vi "Ignition.vi"(7 "Log File Refnum in":refnum<file>, 8 "error in":errorcluster, 9 "UI Data in":T2, 10 "Handshake Notifier in":refnum<notifier>, 11 "Message Queues in":T1) -> (0 "error out":errorcluster, 1 "UI Data out":T2, 2 "Handshake Notifier out":refnum<notifier>, 3 "Message Queues out":T1, 5 "Log File Refnum out":refnum<file>)   [LabVIEW 2014, in "Controller.lvlib"]
doc: "Light the pilot for the boiler."
uses:
  Controller.lvlib
  support/Boiler System Globals.vi
  controls/MHL Status.ctl
  support/Message Queue/Message Cluster.ctl
  support/Message Queue/All Message Queues.ctl
  controls/MHL UI Data.ctl
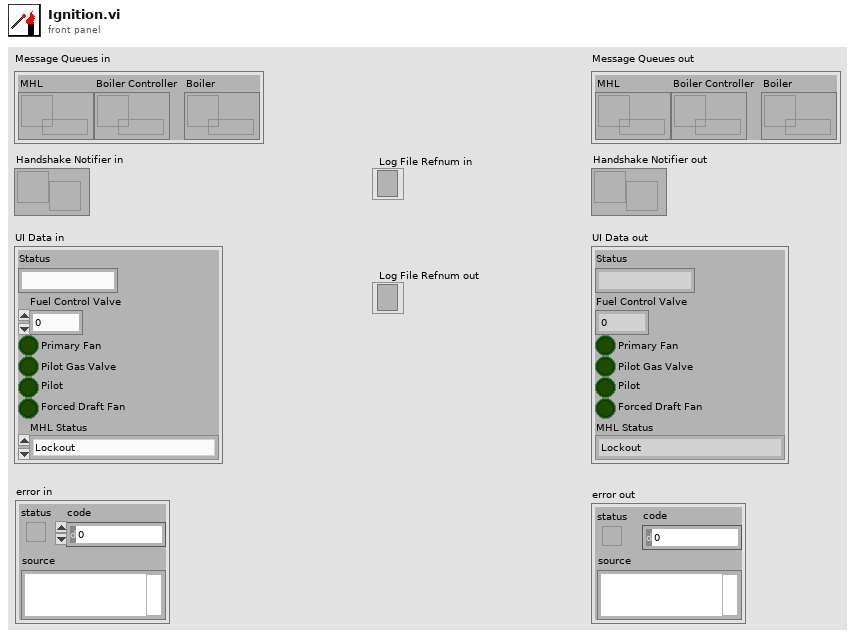
[diagram p1: front panel]
types:
  T1 = typedef "Message Queue.lvlib/All Message Queues.ctl" = cluster{"MHL":refnum<queue>, "Boiler Controller":refnum<queue>, "Boiler":refnum<queue>}
  T2 = typedef "MHL UI Data.ctl" = cluster{"Status":string, "Fuel Control Valve":u32, "Primary Fan":bool, "Pilot Gas Valve":bool, "Pilot":bool, "Forced Draft Fan":bool, "MHL Status":T3}
  T3 = typedef "MHL Status.ctl" = enum16{"Lockout", "Ready", "Pre-Purge", "Pre-Purge Complete", "Pilot On", "Boiler Running", "Shutdown", "Purge"}
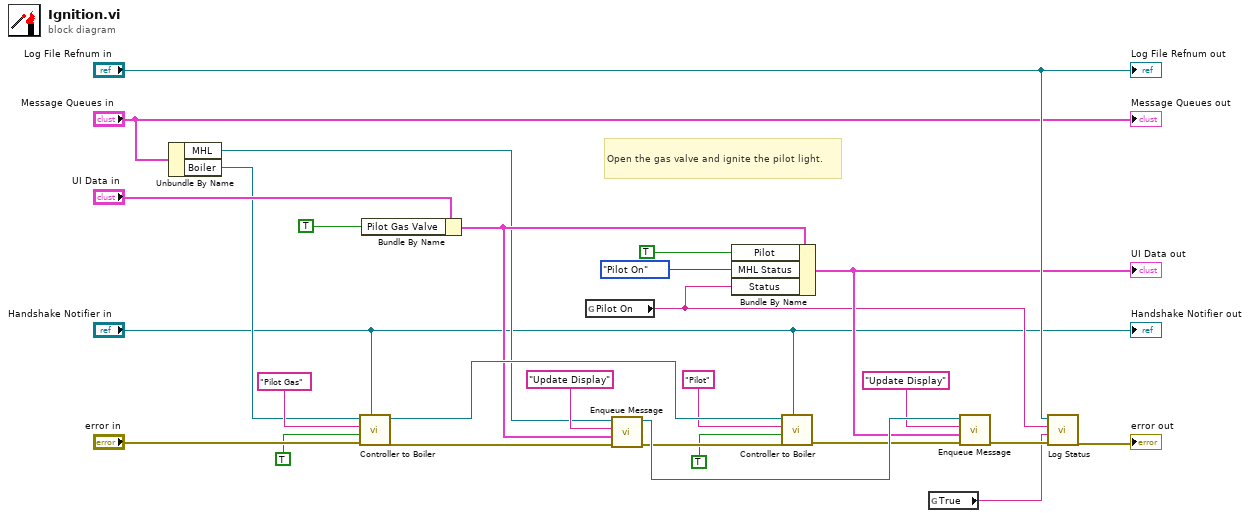
[diagram p0: block diagram]
diagram:
  # "Open the gas valve and ignite the pilot light."
  n1 = Unbundle By Name("Message Queues in") -> ("MHL"=w7:refnum<queue>, "Boiler"=w6:refnum<queue>)
  n2 = call "Controller to Boiler.vi"("Notifier"="Handshake Notifier in", "error in"="error in", "Message Data"=TRUE, "Message"="Pilot Gas", "Boiler Queue in"=w6) -> ("error out"=w22:errorcluster, "Queue out"=w26:refnum<queue>)  [unwired: 4 in, 1 out]
  n3 = Bundle By Name(cluster="UI Data in", "Pilot Gas Valve"=TRUE ("Natural Gas Valve")) -> (w25:T2)
  n4 = global read "Boiler System Globals.vi" "Pilot On"() -> (w4:string)
  n5 = call "Enqueue Message.vi"("error in (no error)"=w22, "Message Data"=w25, "Message"="Update Display", "Message Queue"=w7) -> ("error out"=w21:errorcluster, "dup Message Queue"=w23:refnum<queue>)  [unwired: 6 in]
  n6 = Bundle By Name(cluster=w25, "Pilot"=TRUE, "MHL Status"=MHL_Status."Pilot On", "Status"=w4) -> (w14:T2)
  "UI Data out" <- w14
  n7 = call "Controller to Boiler.vi"("Notifier"="Handshake Notifier in", "error in"=w21, "Message Data"=TRUE, "Message"="Pilot", "Boiler Queue in"=w26) -> ("error out"=w18:errorcluster)  [unwired: 4 in, 2 out]
  n8 = global read "Boiler System Globals.vi" "True"() -> (w3:string)
  n9 = call "Enqueue Message.vi"("error in (no error)"=w18, "Message Data"=w14, "Message"="Update Display", "Message Queue"=w23) -> ("error out"=w9:errorcluster)  [unwired: 6 in, 1 out]
  n10 = call "Log Status.vi"("error in"=w9, "Event Data String (-)"=w3, "Event String"=w4, "Log File Refnum In"="Log File Refnum in") -> ("error out"=→"error out":errorcluster)  [unwired: 6 in, 1 out]
  "Log File Refnum out" <- "Log File Refnum in"
  "Message Queues out" <- "Message Queues in"
  "Handshake Notifier out" <- "Handshake Notifier in"
